vi "Change BD Constant Value.vi"(6 "Assert VI Path":path, 8 "error in (no error)":errorcluster, 9 "Data Value":variant, 10 "Constant Name":string) -> (0 "error out":errorcluster)   [LabVIEW 2016]
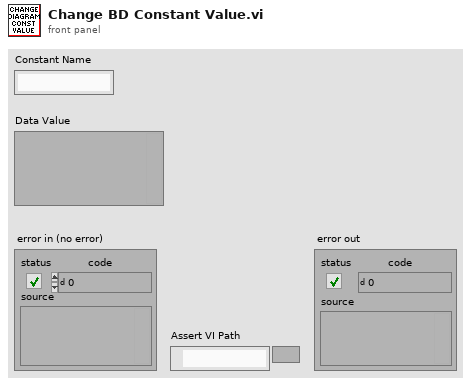
[diagram p1: front panel]
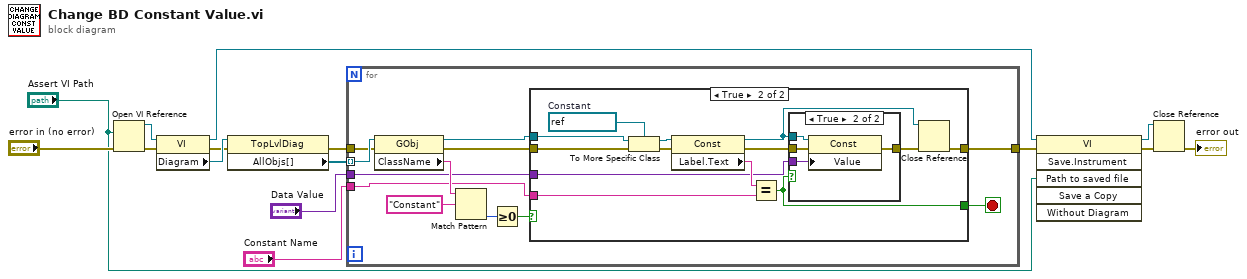
[diagram p0: block diagram]
diagram:
  n1 = Open VI Reference(vi path="Assert VI Path", error in (no error)="error in (no error)") -> (vi reference=w2:refnum<vi>, error out=w1:errorcluster)  [unwired: 4 in]
  n2 = property class="VI"(reference=w2, error in=w1) -> (reference out=w4:refnum<vi>, error out=w14:errorcluster, "Diagram"=w15:refnum<vi>)
  n3 = property class="TopLvlDiag"(reference=w15, error in=w14) -> (error out=w12:errorcluster, "AllObjs[]"=w13:refnum<vi>[])  [unwired: 1 out]
  n4 = for {
    tunnel: w13 -> [w27] mode=indexing
    tunnel: w12 -> [w26]
    tunnel: [w21] -> w3
    tunnel: "Constant Name" -> [w19]
    tunnel: "Data Value" -> [w17]
    stop <- w16 stop-if-true
    n5 = property class="GObj"(reference=w27, error in=w26) -> (reference out=w20:refnum<vi>, error out=w25:errorcluster, "ClassName"=w24:string)
    n6 = Match Pattern(string=w24, regular expression="Constant") -> (offset past match=w22:i32)  [unwired: 1 in, 3 out]
    n7 = Greater Or Equal To 0?(x=w22) -> (x >= 0?=w18:bool)
    n8 = case shown="True" w18 {
      tunnel: w25 -> [w28 w41]
      tunnel: [w28 w32] -> w21
      tunnel: w20 -> [_ w39]
      tunnel: w19 -> [_ w34]
      tunnel: w17 -> [_ w30]
      tunnel: [_ w29] -> w16
      frame False {
      }
      frame True {
        w38 = refnum<vi> refnum  # Constant
        n9 = To More Specific Class(target class=w38, reference=w39, error in=w41) -> (specific class reference=w36:refnum<vi>, error out=w40:errorcluster)
        n10 = property class="Const"(reference=w36, error in=w40) -> (reference out=w31:refnum<vi>, error out=w37:errorcluster, "Label.Text"=w35:string)
        n11 = Equal?(x=w35, y=w34) -> (x = y?=w29:bool)
        n12 = case shown="True" w29 {
          tunnel: w37 -> [w42 w46]
          tunnel: [w42 w45] -> w33
          tunnel: w31 -> [_ w44]
          tunnel: w30 -> [_ w43]
          frame False {
          }
          frame True {
            n13 = property class="Const"(reference=w44, error in=w46, "Value"=w43) -> (error out=w45:errorcluster)  [unwired: 1 out]
          }
        }
        n14 = Close Reference(reference=w31, error in (no error)=w33) -> (error out=w32:errorcluster)
      }
    }
  }
  n15 = invoke class="VI" method="Save.Instrument"(reference=w4, error in=w3, "Path to saved file"="Assert VI Path") -> (reference out=w6:refnum<vi>, error out=w7:errorcluster)  [unwired: 3 in, 4 out]
  n16 = Close Reference(reference=w6, error in (no error)=w7) -> (error out=→"error out":errorcluster)
